vi "Read Keys.vi"(8 "error in (no error)":errorcluster, 11 "Section 1 in":refnum<class "Section 1.lvclass">) -> (0 "error out":errorcluster, 2 "Keys":cluster{"Name":string, "Value":string}[](array[cluster]), 3 "Section 1 out":refnum<class "Section 1.lvclass">)   [LabVIEW 2016, in "LVOOP Introduction.lvlib" / "Section 1.lvclass"]
doc: "Thi VI returns an array of key/values pairs of section.\n\nOverwriting dynamic dispatch VI."
uses:
  Section 1.lvclass
  Read Boolean.vi
  Read Double.vi
  Read String.vi
  Configuration/Classes/Section/Section.lvclass
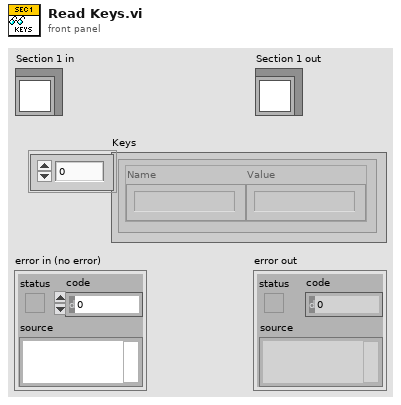
[diagram p1: front panel]
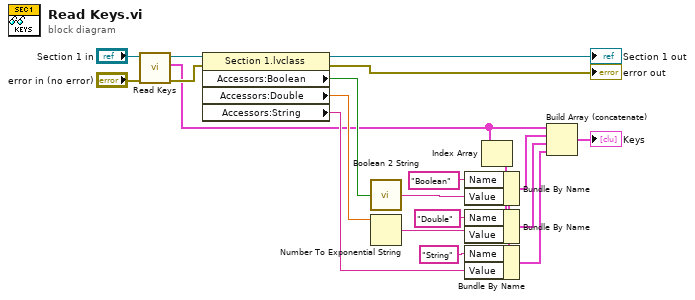
[diagram p0: block diagram]
diagram:
  n1 = call-parent "Read Keys.vi"("error in (no error)"="error in (no error)", "Section in"="Section 1 in") -> ("error out"=w17:errorcluster, "Keys"=w5:cluster{"Name":string, "Value":string}[], "Section out"=w15:refnum<class "Section 1.lvclass">)  [unwired: 7 in]
  n2 = property class="Section 1.lvclass"(reference=w15, error in=w17) -> (reference out=→"Section 1 out":refnum<class "Section 1.lvclass">, error out=→"error out":errorcluster, "Accessors:Boolean"=w12:bool, "Accessors:Double"=w7:dbl, "Accessors:String"=w8:string)
  n3 = call "Boolean 2 String.vi"("Boolean"=w12) -> ("Boolean String"=w11:string)
  n4 = Number To Exponential String(number=w7) -> (E-format string=w6:string)  [unwired: 3 in]
  n5 = Index Array(array=w5) -> (element=w18:cluster{"Name":string, "Value":string})  [unwired: 1 in]
  n6 = Bundle By Name(cluster=w18, "Name"="String", "Value"=w8) -> (w2:cluster{"Name":string, "Value":string})
  n7 = Bundle By Name(cluster=w2, "Name"="Double", "Value"=w6) -> (w3:cluster{"Name":string, "Value":string})
  n8 = Bundle By Name(cluster=w3, "Name"="Boolean", "Value"=w11) -> (w4:cluster{"Name":string, "Value":string})
  n9 = Build Array (concatenate)(w5, w4, w3, w2) -> (→"Keys":cluster{"Name":string, "Value":string}[])
